vi "save_file.vi"(5 "write OME header?":bool, 7 "path":path, 8 "error in (no error)":errorcluster, 10 "ImageCollection in":refnum<class "ImageCollection.lvclass">=refnum, 11 "DataCollectionDL090215 in":refnum<class "DataCollectionDL091104Scaffold.lvclass">) -> (0 "error out":errorcluster, 3 "DataCollectionDL090215 out":refnum<class "DataCollectionDL091104Scaffold.lvclass">)   [LabVIEW 2010]
uses:
  DataCollectionDL091104Scaffold.lvclass
  bricks/classes/ImageCollection/ImageCollection.lvclass
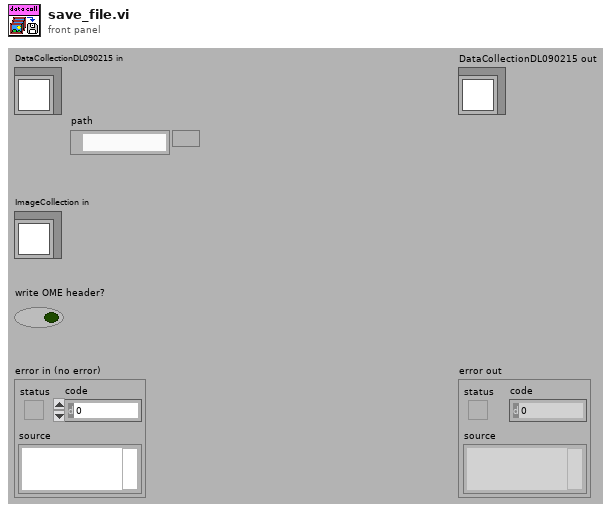
[diagram p1: front panel]
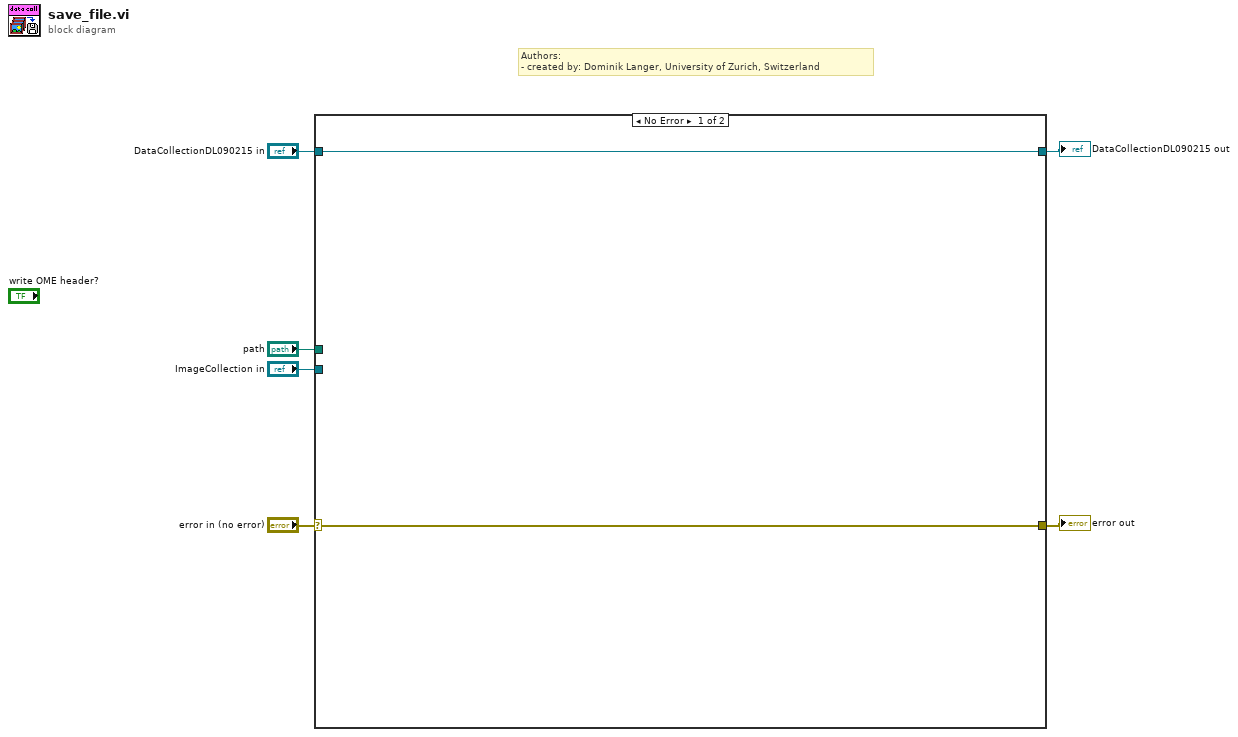
[diagram p0: block diagram]
diagram:
  # "Authors: \n- created by: Dominik Langer, University of Zurich, Switzerland"
  n1 = case shown="No Error" "error in (no error)" {
    selector: "error in (no error)" -> [w7 w10]
    tunnel: [w7 w10] -> w5
    tunnel: [w8 w9] -> w3
    tunnel: "DataCollectionDL090215 in" -> [w8 w9]
    tunnel: "path" -> [_ _]
    tunnel: "ImageCollection in" -> [_ _]
    frame No Error {
    }
    frame Error {
    }
  }
  "error out" <- w5
  "DataCollectionDL090215 out" <- w3
